vi "Data File Processing UI Build Type Nodata Messages.vi"(7 "type":T1) -> (8 "msg out":T2[](array[typedef]))   [LabVIEW 2012]
uses:
  Data File Processing UI Message Define.ctl
  Data File Processing UI Message Type Define.ctl
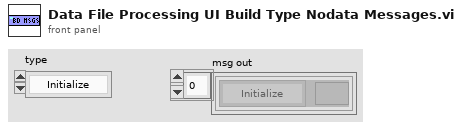
[diagram p1: front panel]
types:
  T1 = typedef "Data File Processing UI Message Type Define.ctl" = enum32{"Initialize", "SleepThread", "ErrorHandler", "NoEvent", "PreExit", "Exit", "----Action----", "OpenFile", "ReadAllCompute", "SaveFile", "RedrawGraph", "SelectChannel"}
  T2 = typedef "Data File Processing UI Message Define.ctl" = cluster{"data":variant, "type":T1}
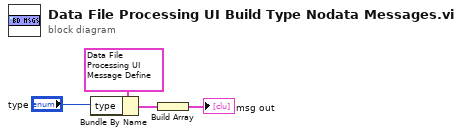
[diagram p0: block diagram]
diagram:
  n1 = Bundle By Name(cluster=T2 {"data"=variant, "type"=enum."Initialize"} ("MsgDef"), "type"="type") -> (w3:T2)
  n2 = Build Array(w3) -> (→"msg out":T2[])
